vi "ProcessValues.vi"(11 "ArrayIn":u8[](array[numeric])) -> ()   [LabVIEW 2011]
uses:
  Strict Type Controls/Settings Operation.ctl
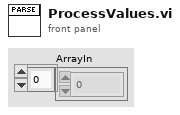
[diagram p1: front panel]
types:
  T1 = typedef "Settings Operation.ctl" = enum8{"Get Value", "Set Value", "Read File", "Write File", "Write Stored Value"}
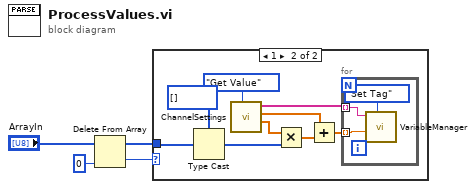
[diagram p0: block diagram]
diagram:
  n1 = Delete From Array(array="ArrayIn", index=0) -> (deleted portion=w3:u8, array with subset deleted=w4:u8[])  [unwired: 1 in]
  n2 = case shown="1" w3 {
    tunnel: w4 -> [_ w13]
    frame 0, Default {
    }
    frame 1 {
      n3 = Type Cast(type=u16[] [], x=w13) -> (*(type *) &x=w11:u16[])
      n4 = call "ChannelSettings.vi"("Operation"=Settings_Operation."Get Value") -> ("Scale"=w5:dbl[], "Offset"=w6:dbl[], "Name"=w7:string[])  [unwired: 5 in, 2 out]
      n5 = Multiply(x=w5, y=w11) -> (x*y=w10:dbl[])
      n6 = Add(x=w6, y=w10) -> (x+y=w8:dbl[])
      n7 = for {
        tunnel: w8 -> [w16] mode=indexing
        tunnel: w7 -> [w15] mode=indexing
        n8 = call "VariableManager.vi"("Operation"=enum16{"Get Tag", "Set Tag"}."Set Tag", "Value"=w16, "Tag"=w15) -> ()  [unwired: 9 out]
      }
    }
  }
